vi "WriteL.vi"(8 "error in (no error)":errorcluster, 9 "val":u32, 10 "offset":u32) -> (0 "error out":errorcluster)   [LabVIEW 2015, in "ESLSCDLL.lvlib"]
uses:
  ESLSCDLL.lvlib
  Globals.vi
  ESLSCDLL.dll
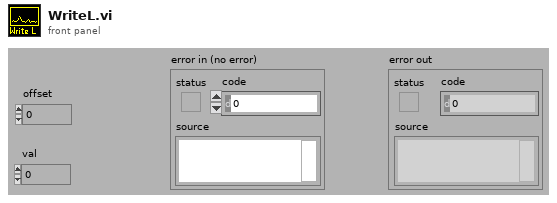
[diagram p1: front panel]
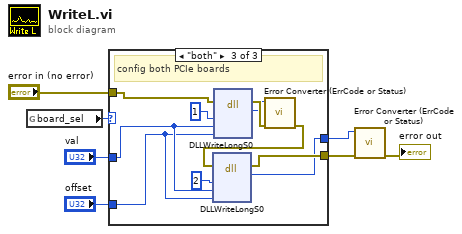
[diagram p0: block diagram]
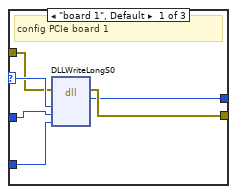
[diagram p2: hidden frame]
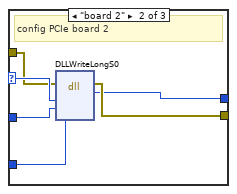
[diagram p3: hidden frame]
diagram:
  n1 = global read "Globals.vi" "board_sel"() -> (w1:enum32{"0", "board 1", "board 2", "both"})
  n2 = case shown="\"both\"" w1 {
    selector: w1 -> [w13 w19 _]
    tunnel: "val" -> [w12 w18 w27]
    tunnel: "offset" -> [w11 w17 w26]
    tunnel: "error in (no error)" -> [w10 w14 w25]
    tunnel: [w9 w16 w21] -> w3
    tunnel: [w8 w15 w20] -> w2
    frame "board 1", Default {
      # "config PCIe board 1"
      n3 = dll-call lib="C:/ENTW/PCIE/LV64/board.vis/ESLSCDLL.dll" fn="DLLWriteLongS0"(error in=w10, "drv"=w13, "DataByte"=w12, "PortOff"=w11) -> (error out=w9:errorcluster, "es_status_codes"=w8:i32)  [unwired: 5 in, 1 out]
    }
    frame "board 2" {
      # "config PCIe board 2"
      n4 = dll-call lib="C:/ENTW/PCIE/LV64/board.vis/ESLSCDLL.dll" fn="DLLWriteLongS0"(error in=w14, "drv"=w19, "DataByte"=w18, "PortOff"=w17) -> (error out=w16:errorcluster, "es_status_codes"=w15:i32)  [unwired: 5 in, 1 out]
    }
    frame "both" {
      # "config both PCIe boards"
      n5 = dll-call lib="C:/ENTW/PCIE/LV64/board.vis/ESLSCDLL.dll" fn="DLLWriteLongS0"(error in=w25, "drv"=u32 1, "DataByte"=w27, "PortOff"=w26) -> (error out=w24:errorcluster, "es_status_codes"=w23:i32)  [unwired: 5 in, 1 out]
      n6 = call "Error Converter (ErrCode or Status).vi"("error in (no error)"=w24, "error code"=w23) -> ("error out"=w22:errorcluster)  [unwired: 9 in]
      n7 = dll-call lib="C:/ENTW/PCIE/LV64/board.vis/ESLSCDLL.dll" fn="DLLWriteLongS0"(error in=w22, "drv"=u32 2, "DataByte"=w27, "PortOff"=w26) -> (error out=w21:errorcluster, "es_status_codes"=w20:i32)  [unwired: 5 in, 1 out]
    }
  }
  n8 = call "Error Converter (ErrCode or Status).vi"("error in (no error)"=w3, "error code"=w2) -> ("error out"=→"error out":errorcluster)  [unwired: 9 in]
